vi "Read All Elements GUI.vi"(8 "error in (no error)":errorcluster, 11 "Storage params in":refnum<class "CV-Storage.lvclass">) -> (0 "error out":errorcluster, 2 "Storage params.":T1={"Base file name"="Test", "Storage directory"=path "C:/CameraVision/Results", "Save what?"={"Original"=FALSE, "Corrected"=FALSE, "Binary"=FALSE, "Temperature"=FALSE, "Characteristics"=FALSE, "Mapping"=FALSE, "TemperatureValues"=FALSE}, "Image file type"=enum."BMP", "Comments"="", "Storage mode"=enum."1 file for all layers ", "Start iteration/layer"=0}, 3 "Storage params out":refnum<class "CV-Storage.lvclass">)   [LabVIEW 2013, in "CameraVision.lvlib" / "CV-Storage.lvclass"]
uses:
  CV-Storage.lvclass
  Storage-parameters-gui.ctl
  Storage-types.ctl
  CV-Storage.lvclass/CV-Storage.ctl
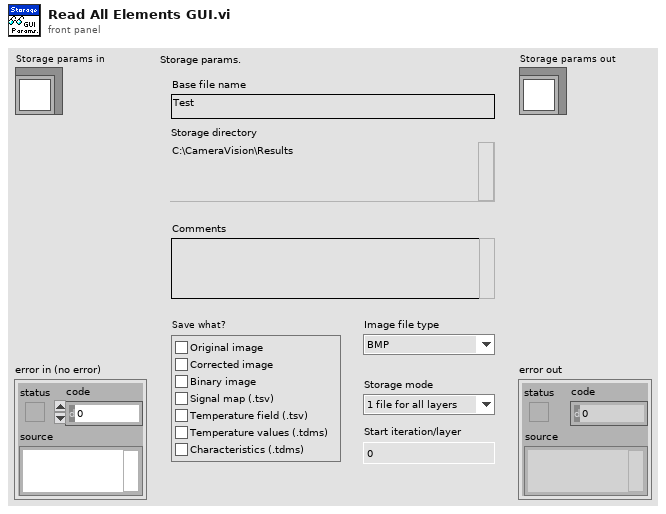
[diagram p1: front panel]
types:
  T1 = typedef "CameraVision.lvlib/CV-Storage.lvclass/Storage-parameters-gui.ctl" = cluster{"Base file name":string, "Storage directory":path, "Save what?":T2, "Image file type":enum16{"JPG", "BMP", "PNG"}, "Comments":string, "Storage mode":enum16{"1 file per layer", "1 file for all layers "}, "Start iteration/layer":u16}
  T2 = typedef "CameraVision.lvlib/CV-Storage.lvclass/Storage-types.ctl" = cluster{"Original":bool, "Corrected":bool, "Binary":bool, "Temperature":bool, "Characteristics":bool, "Mapping":bool, "TemperatureValues":bool}
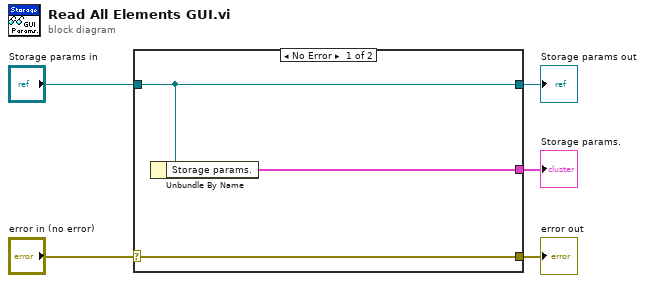
[diagram p0: block diagram]
diagram:
  n1 = case shown="No Error" "error in (no error)" {
    selector: "error in (no error)" -> [w8 w9]
    tunnel: [w8 w9] -> w4
    tunnel: [w7 w10] -> w2
    tunnel: "Storage params in" -> [w7 w10]
    tunnel: [w6 _] -> w1
    frame No Error {
      n2 = Unbundle By Name(w7) -> ("Storage params."=w6:T1)
    }
    frame Error {
    }
  }
  "error out" <- w4
  "Storage params out" <- w2
  "Storage params." <- w1
